vi "Data Changed__ogtk.vi"   [LabVIEW 2020]
doc: "<B>Data Changed</B>\nThis is a polymorphic VI that will output a true if the data flowing into it has changed. It is also a Reentrant VI. So each intance of it in your code is treated as a seperate VI. The first time that the VI is run it will output a false. It can take any data type as an input. It has several native data types (for efficiency) and will coerce to variant if a non-native data type (error cluster, refnum, etc) is used."
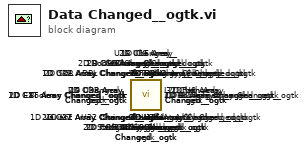
[diagram p0: block diagram]
diagram:
  n1 = call <userlib>:"String Changed__ogtk.vi"() -> ()  [unwired: 1 in, 1 out]
  n2 = call <userlib>:"EXT Changed__ogtk.vi"() -> ()  [unwired: 1 in, 1 out]
  n3 = call <userlib>:"Boolean Changed__ogtk.vi"() -> ()  [unwired: 1 in, 1 out]
  n4 = call <userlib>:"CDB Changed__ogtk.vi"() -> ()  [unwired: 1 in, 1 out]
  n5 = call <userlib>:"CSG Changed__ogtk.vi"() -> ()  [unwired: 1 in, 1 out]
  n6 = call <userlib>:"CXT Changed__ogtk.vi"() -> ()  [unwired: 1 in, 1 out]
  n7 = call <userlib>:"DBL Changed__ogtk.vi"() -> ()  [unwired: 1 in, 1 out]
  n8 = call <userlib>:"I16 Changed__ogtk.vi"() -> ()  [unwired: 1 in, 1 out]
  n9 = call <userlib>:"I32 Changed__ogtk.vi"() -> ()  [unwired: 1 in, 1 out]
  n10 = call <userlib>:"I8 Changed__ogtk.vi"() -> ()  [unwired: 1 in, 1 out]
  n11 = call <userlib>:"SGL Changed__ogtk.vi"() -> ()  [unwired: 1 in, 1 out]
  n12 = call <userlib>:"U16 Changed__ogtk.vi"() -> ()  [unwired: 1 in, 1 out]
  n13 = call <userlib>:"U32 Changed__ogtk.vi"() -> ()  [unwired: 1 in, 1 out]
  n14 = call <userlib>:"Variant Changed__ogtk.vi"() -> ()  [unwired: 1 in, 1 out]
  n15 = call <userlib>:"U8 Changed__ogtk.vi"() -> ()  [unwired: 1 in, 1 out]
  n16 = call <userlib>:"1D Boolean Array Changed__ogtk.vi"() -> ()  [unwired: 1 in, 1 out]
  n17 = call <userlib>:"1D CDB Array Changed__ogtk.vi"() -> ()  [unwired: 1 in, 1 out]
  n18 = call <userlib>:"1D CSG Array Changed__ogtk.vi"() -> ()  [unwired: 1 in, 1 out]
  n19 = call <userlib>:"1D CXT Array Changed__ogtk.vi"() -> ()  [unwired: 1 in, 1 out]
  n20 = call <userlib>:"2D Variant Array Changed__ogtk.vi"() -> ()  [unwired: 1 in, 1 out]
  n21 = call <userlib>:"1D Variant Array Changed__ogtk.vi"() -> ()  [unwired: 1 in, 1 out]
  n22 = call <userlib>:"2D String Array Changed__ogtk.vi"() -> ()  [unwired: 1 in, 1 out]
  n23 = call <userlib>:"2D U8 Array Changed__ogtk.vi"() -> ()  [unwired: 1 in, 1 out]
  n24 = call <userlib>:"2D U32 Array Changed__ogtk.vi"() -> ()  [unwired: 1 in, 1 out]
  n25 = call <userlib>:"2D Path Array Changed__ogtk.vi"() -> ()  [unwired: 1 in, 1 out]
  n26 = call <userlib>:"2D U16 Array Changed__ogtk.vi"() -> ()  [unwired: 1 in, 1 out]
  n27 = call <userlib>:"2D SGL Array Changed__ogtk.vi"() -> ()  [unwired: 1 in, 1 out]
  n28 = call <userlib>:"2D I8 Array Changed__ogtk.vi"() -> ()  [unwired: 1 in, 1 out]
  n29 = call <userlib>:"2D I32 Array Changed__ogtk.vi"() -> ()  [unwired: 1 in, 1 out]
  n30 = call <userlib>:"2D I16 Array Changed__ogtk.vi"() -> ()  [unwired: 1 in, 1 out]
  n31 = call <userlib>:"2D DBL Array Changed__ogtk.vi"() -> ()  [unwired: 1 in, 1 out]
  n32 = call <userlib>:"2D EXT Array Changed__ogtk.vi"() -> ()  [unwired: 1 in, 1 out]
  n33 = call <userlib>:"2D CXT Array Changed__ogtk.vi"() -> ()  [unwired: 1 in, 1 out]
  n34 = call <userlib>:"1D String Array Changed__ogtk.vi"() -> ()  [unwired: 1 in, 1 out]
  n35 = call <userlib>:"2D CSG Array Changed__ogtk.vi"() -> ()  [unwired: 1 in, 1 out]
  n36 = call <userlib>:"2D CDB Array Changed__ogtk.vi"() -> ()  [unwired: 1 in, 1 out]
  n37 = call <userlib>:"2D Boolean Array Changed__ogtk.vi"() -> ()  [unwired: 1 in, 1 out]
  n38 = call <userlib>:"1D U8 Array Changed__ogtk.vi"() -> ()  [unwired: 1 in, 1 out]
  n39 = call <userlib>:"1D U32 Array Changed__ogtk.vi"() -> ()  [unwired: 1 in, 1 out]
  n40 = call <userlib>:"1D U16 Array Changed__ogtk.vi"() -> ()  [unwired: 1 in, 1 out]
  n41 = call <userlib>:"1D SGL Array Changed__ogtk.vi"() -> ()  [unwired: 1 in, 1 out]
  n42 = call <userlib>:"1D I8 Array Changed__ogtk.vi"() -> ()  [unwired: 1 in, 1 out]
  n43 = call <userlib>:"1D I16 Array Changed__ogtk.vi"() -> ()  [unwired: 1 in, 1 out]
  n44 = call <userlib>:"1D I32 Array Changed__ogtk.vi"() -> ()  [unwired: 1 in, 1 out]
  n45 = call <userlib>:"1D EXT Array Changed__ogtk.vi"() -> ()  [unwired: 1 in, 1 out]
  n46 = call <userlib>:"1D DBL Array Changed__ogtk.vi"() -> ()  [unwired: 1 in, 1 out]
  n47 = call <userlib>:"1D Path Array Changed__ogtk.vi"() -> ()  [unwired: 1 in, 1 out]
